vi "Outputs SW Set.vi"(6 "CMD_ACT_Tempplate Data":T1, 7 "Current Time":timestamp format="%<%x %.3X>T", 8 "HW Config":T4={"Ver"=0, "CAN"={"ID"=0, "Bus"=""}, "Output"={"Type"=enum."Counter-Clockwise", "Neutral"=enum."Override to Coast", "Max"={"FWD"=1.0, "REV"=-1.0}, "Min"={"FWD"=0.0, "REV"=0.0}, "OL Ramp Rate (S)"=0.0, "Dead Band"=0.0, "CL Ramp Rate (S)"=0.0}, "CL"={"Gains"={"P"=1.0, "I"=0.01, "D"=0.0, "F"=0.0}, "Error Allowed"=0.0, "I Zone"=0.0, "Peak Out 0-1"=10000.0, "Max I Accu"=-1000.0}, "MM"={"Cruise Velocity"=5000, "Acceleration"=5000}, "TravelLimits"={"Hard"={"FWD Switch Normal"=enum."Normally Open", "FWD On will Zero Encoder "=FALSE, "REV Switch Normal"=enum."Normally Open", "REV On will Zero Encoder "=FALSE}, "Soft"={"FWD"={"Enable"=FALSE, "Counts"=0}, "REV"={"Enable"=FALSE, "Counts"=0}}}, "CurrentLimit"={"Enable"=FALSE, "Current Limit"=0.0, "Threshold Current"=0.0, "Threshold Time"=0.0}} {"CL"."Gains"."F" format="%#.8f"; "CL"."Gains"."D" format="%#.8f"; "CL"."Gains"."I" format="%#.8f"; "CL"."Gains"."P" format="%#.8f"; "Output"."Min"."REV" format="%.2f"; "Output"."Min"."FWD" format="%.2f"; "Output"."Max"."REV" format="%.2f"; "Output"."Max"."FWD" format="%.2f"; "TravelLimits"."Soft"."REV"."Counts" format="%#.0f"; "TravelLimits"."Soft"."FWD"."Counts" format="%#.0f"}, 9 "SW Config":T19={"Ver"=0, "Pivot Arm Position Table"={"Full Back"=0.2, "Full Forward"=0.0, "Amp Score"=0.0, "Pivot Arm Load"=0.0, "Vertical"=0.0, "Trap Score"=0.0}}, 10 "Sensor Values":T22 {"Set"."Mode" items=["PercentOutput"=0, "Position"=1, "Velocity"=2, "Current"=3, "Follower"=5, "MotionProfile"=6, "MotionMagic"=7, "MotionProfileArc"=10, "Disabled"=15]}, 11 "SW Output":T21) -> (3 "SW Output Out":T21)   [LabVIEW 2023, in "Shooter FX_ACT.lvlib"]
uses:
  Shooter FX_ACT.lvlib
  Shared Code/TypeDefs/Cluster_FX Sensor Values.ctl
  Shared Code/TypeDefs/Cluster_FX CloseLoop Values.ctl
  Shared Code/TypeDefs/Cluster_FX Limit Switchs.ctl
  Shared Code/TypeDefs/Cluster_FX Current Values.ctl
  Cluster_HW Output Values.ctl
  Cluster_SW Output Data.ctl
  Cluster_Config SW Values.ctl
  Shared Code/TypeDefs/Cluster_FWD  REV Values.ctl
  Shared Code/TypeDefs/Cluster_PID Gains.ctl
  Shared Code/TypeDefs/Cluster_FX Motion Magic Parameters.ctl
  Shared Code/TypeDefs/Cluser_CAN Data.ctl
  <vilib>/Rock Robotics/WPI/ThirdParty/Phoenix-LabVIEW/Motor Controller/Controls/CTRE_Phoenix_MotorControl_NeutralMode.ctl
  <vilib>/Rock Robotics/WPI/ThirdParty/Phoenix-LabVIEW/Motor Controller/Controls/CTRE_Phoenix_MotorControl_LimitSwitchNormal.ctl
  Shared Code/TypeDefs/Cluser_Hard Limits.ctl
  Shared Code/TypeDefs/Cluser_Enable-Value I32.ctl
  Shared Code/TypeDefs/Cluser_Config_Soft Limits.ctl
  Shared Code/TypeDefs/Cluser_FX Config_Limit Travel.ctl
  Cluster_Config HW Values.ctl
  Shared Code/TypeDefs/Cluser_FX Config_Current Limits.ctl
  Shared Code/TypeDefs/Cluster_FX_HW All Sensor Values.ctl
  <vilib>/Rock Robotics/WPI/ThirdParty/Phoenix-LabVIEW/Motor Controller/Controls/CTRE_Phoenix_MotorControl_ControlMode.ctl
  Shared Code/TypeDefs/Cluster_FX Output Set Values.ctl
  <vilib>/Rock Robotics/WPI/ThirdParty/Phoenix-LabVIEW/Motor Controller/Controls/CTRE_Phoenix_MotorControl_TalonFXInvertType.ctl
  Shared Code/TypeDefs/Cluster_Config FX Motor Output.ctl
  Shared Code/TypeDefs/Cluster_FX SLOT PID Config.ctl
  Shared Code/TypeDefs/Cluster_Pivot Arm Position Table.ctl
  ENUM_CMD_Mode Select.ctl
  Shared Code/TypeDefs/ENUM_Pivot Arm Position Select.ctl
  Cluster_CMD_ACT_Data.ctl
panel:
  # "Tune Output\nto 1023 Max"
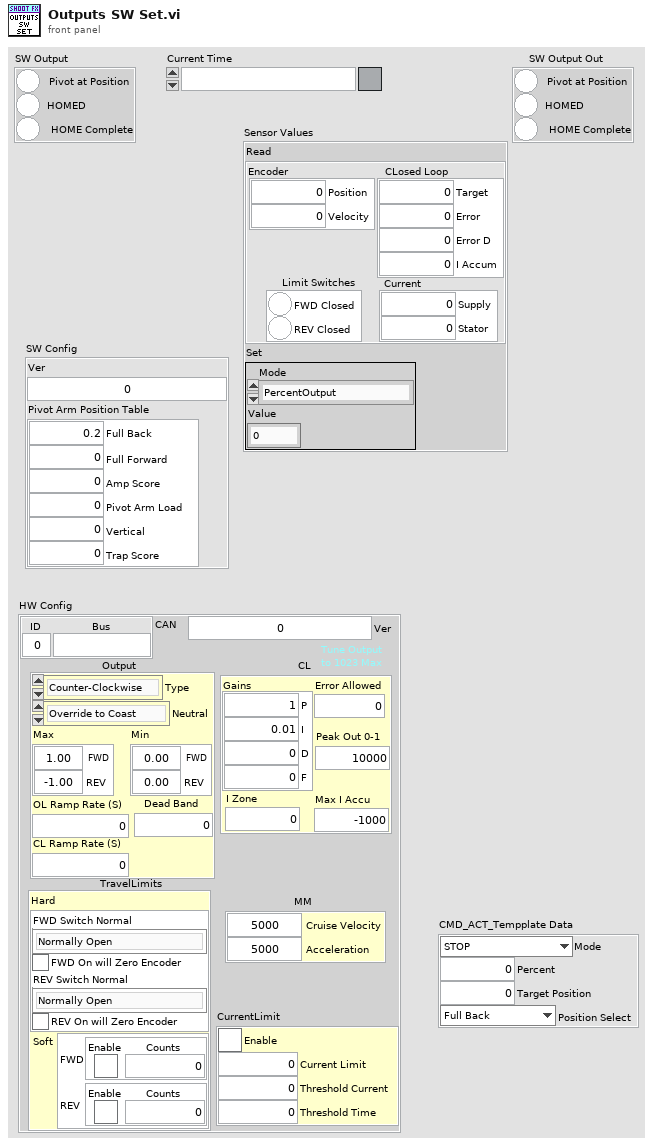
[diagram p1: front panel]
types:
  T1 = typedef "Shooter FX_ACT.lvlib/Cluster_CMD_ACT_Data.ctl" = cluster{"Mode":T2, "Percent":dbl, "Target Position":dbl, "Position Select":T3}
  T2 = typedef "Shooter FX_ACT.lvlib/ENUM_CMD_Mode Select.ctl" = enum16{"STOP", "PercentOut", "Positon Value", "Position Select"}
  T3 = typedef "ENUM_Pivot Arm Position Select.ctl" = enum16{"Full Back", "Full Forward", "Amp Score", "Pivot Arm Load", "Vertical", "Trap Score"}
  T4 = typedef "Shooter FX_ACT.lvlib/Cluster_Config HW Values.ctl" = cluster{"Ver":u64, "CAN":T5, "Output":T6, "CL":T10, "MM":T12, "TravelLimits":T13, "CurrentLimit":T18}
  T5 = typedef "Cluser_CAN Data.ctl" = cluster{"ID":u8, "Bus":string}
  T6 = typedef "Cluster_Config FX Motor Output.ctl" = cluster{"Type":T7, "Neutral":T8, "Max":T9, "Min":T9, "OL Ramp Rate (S)":dbl, "Dead Band":dbl, "CL Ramp Rate (S)":dbl}
  T7 = typedef "CTRE_Phoenix_MotorControl_TalonFXInvertType.ctl" = enum16{"Counter-Clockwise", "Clockwise"}
  T8 = typedef "CTRE_Phoenix_MotorControl_NeutralMode.ctl" = enum8{"EEPROMSetting", "Override to Coast", "Override to Brake"}
  T9 = typedef "Cluster_FWD  REV Values.ctl" = cluster{"FWD":dbl, "REV":dbl}
  T10 = typedef "Cluster_FX SLOT PID Config.ctl" = cluster{"Gains":T11, "Error Allowed":dbl, "I Zone":dbl, "Peak Out 0-1":dbl, "Max I Accu":dbl}
  T11 = typedef "Cluster_PID Gains.ctl" = cluster{"P":dbl, "I":dbl, "D":dbl, "F":dbl}
  T12 = typedef "Cluster_FX Motion Magic Parameters.ctl" = cluster{"Cruise Velocity":i32, "Acceleration":i32}
  T13 = typedef "Cluser_FX Config_Limit Travel.ctl" = cluster{"Hard":T14, "Soft":T16}
  T14 = typedef "Cluser_Hard Limits.ctl" = cluster{"FWD Switch Normal":T15, "FWD On will Zero Encoder ":bool, "REV Switch Normal":T15, "REV On will Zero Encoder ":bool}
  T15 = typedef "CTRE_Phoenix_MotorControl_LimitSwitchNormal.ctl" = enum16{"Normally Open", "Normally Closed", "Disabled"}
  T16 = typedef "Cluser_Config_Soft Limits.ctl" = cluster{"FWD":T17, "REV":T17}
  T17 = typedef "Cluser_Enable-Value I32.ctl" = cluster{"Enable":bool, "Counts":i32}
  T18 = typedef "Cluser_FX Config_Current Limits.ctl" = cluster{"Enable":bool, "Current Limit":dbl, "Threshold Current":dbl, "Threshold Time":dbl}
  T19 = typedef "Shooter FX_ACT.lvlib/Cluster_Config SW Values.ctl" = cluster{"Ver":u64, "Pivot Arm Position Table":T20}
  T20 = typedef "Cluster_Pivot Arm Position Table.ctl" = cluster{"Full Back":dbl, "Full Forward":dbl, "Amp Score":dbl, "Pivot Arm Load":dbl, "Vertical":dbl, "Trap Score":dbl}
  T21 = typedef "Shooter FX_ACT.lvlib/Cluster_SW Output Data.ctl" = cluster{"Pivot at Position":bool, "HOMED":bool, "HOME Complete":bool}
  T22 = typedef "Shooter FX_ACT.lvlib/Cluster_HW Output Values.ctl" = cluster{"Read":T23, "Set":T28}
  T23 = typedef "Cluster_FX_HW All Sensor Values.ctl" = cluster{"Encoder":T24, "CLosed Loop":T25, "Limit Switches":T26, "Current":T27}
  T24 = typedef "Cluster_FX Sensor Values.ctl" = cluster{"Position":i32, "Velocity":i32}
  T25 = typedef "Cluster_FX CloseLoop Values.ctl" = cluster{"Target":dbl, "Error":i32, "Error D":dbl, "I Accum":dbl}
  T26 = typedef "Cluster_FX Limit Switchs.ctl" = cluster{"FWD Closed":bool, "REV Closed":bool}
  T27 = typedef "Cluster_FX Current Values.ctl" = cluster{"Supply":dbl, "Stator":dbl}
  T28 = typedef "Cluster_FX Output Set Values.ctl" = cluster{"Mode":T29, "Value":dbl}
  T29 = typedef "CTRE_Phoenix_MotorControl_ControlMode.ctl" = u16
  T30 = cluster{"Start Time":timestamp, "Prev AT Target Pos":bool, "Home Complete":bool}
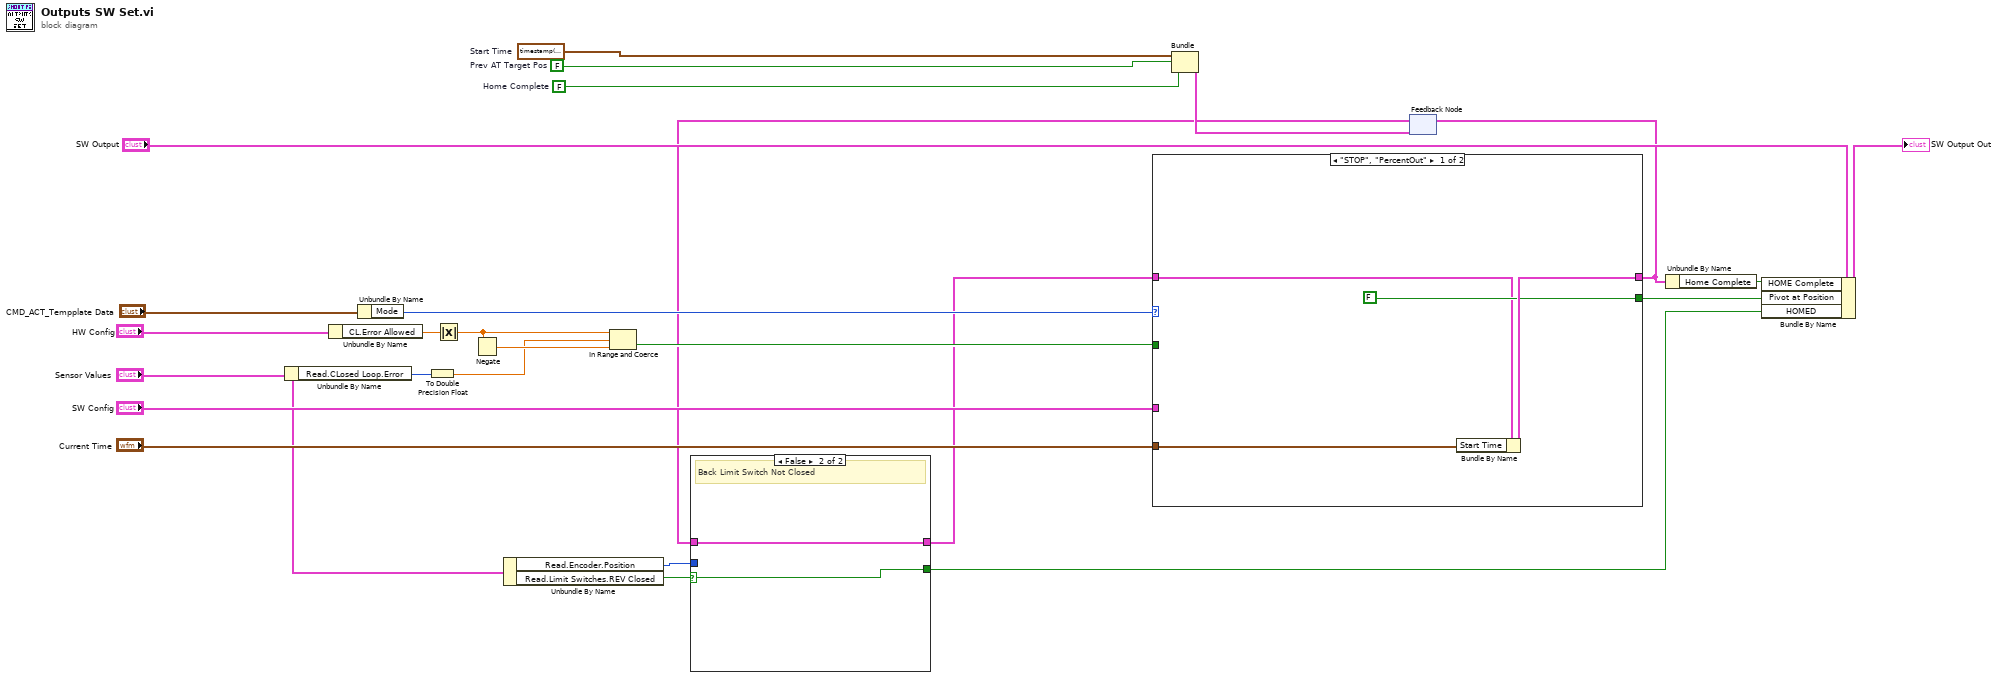
[diagram p0: block diagram]
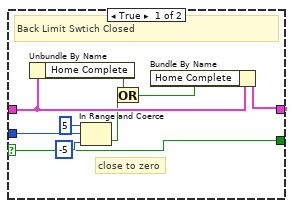
[diagram p2: hidden frame]
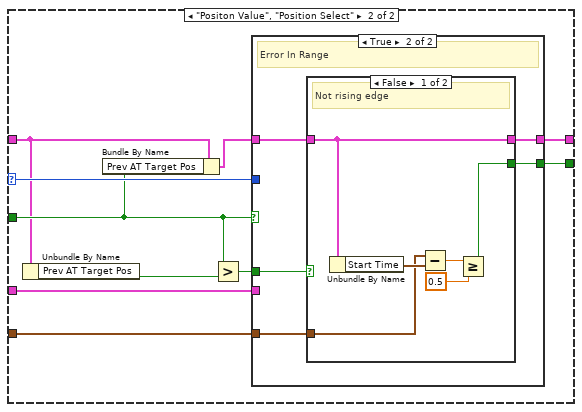
[diagram p3: hidden frame]
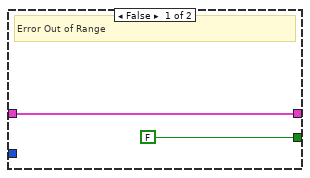
[diagram p4: hidden frame]
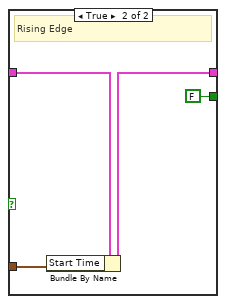
[diagram p5: hidden frame]
diagram:
  w5 = FALSE  # Home Complete
  w10 = FALSE  # Prev AT Target Pos
  w24 = timestamp(0 s since 1904-01-01)  # Start Time
  n1 = Unbundle By Name("Sensor Values") -> ("Read.CLosed Loop.Error"=w19:i32)
  n2 = Unbundle By Name("HW Config") -> ("CL.Error Allowed"=w17:dbl)
  n3 = Unbundle By Name("CMD_ACT_Tempplate Data") -> ("Mode"=w11:T2)
  n4 = To Double Precision Float(number=w19) -> (double precision float=w13:dbl)
  n5 = Absolute Value(x=w17) -> (abs(x)=w16:dbl)
  n6 = Negate(x=w16) -> (-x=w15:dbl)
  n7 = Unbundle By Name("Sensor Values") -> ("Read.Encoder.Position"=w7:i32, "Read.Limit Switches.REV Closed"=w8:bool)
  n8 = In Range and Coerce(upper limit=w16, x=w13, lower limit=w15) -> (In Range?=w18:bool)  [unwired: 1 out]
  n9 = Bundle("Start Time"=w24, "Prev AT Target Pos"=w10, "Home Complete"=w5) -> (w23:T30)  [unwired: 1 in]
  n10 = feedback #1(w23) -> (w4:T30)
  n11 = case shown="False" w8 {
    selector: w8 -> [w28 w37]
    tunnel: w7 -> [w34 _]
    tunnel: [w28 w37] -> w6
    tunnel: w4 -> [w33 w36]
    tunnel: [w35 w36] -> w3
    frame True {
      # "close to zero"
      # "Back Limit Swtich Closed"
      n12 = Unbundle By Name(w33) -> ("Home Complete"=w29:bool)
      n13 = In Range and Coerce(upper limit=5, x=w34, lower limit=-5 ("upper limit")) -> (In Range?=w27:bool)  [unwired: 1 out]
      n14 = Or(x=w29, y=w27) -> (x .or. y?=w30:bool)
      n15 = Bundle By Name(cluster=w33, "Home Complete"=w30) -> (w35:T30)
    }
    frame False {
      # "Back Limit Switch Not Closed"
    }
  }
  n16 = case shown="\"STOP\", \"PercentOut\"" w11 {
    selector: w11 -> [_ w47]
    tunnel: "SW Config" -> [_ w51]
    tunnel: "Current Time" -> [w41 w50]
    tunnel: [w40 w49] -> w2
    tunnel: w18 -> [_ w44]
    tunnel: [FALSE ("Out Data 1") w48] -> w14
    tunnel: w3 -> [w38 w42]
    frame "STOP", "PercentOut" {
      n17 = Bundle By Name(cluster=w38, "Start Time"=w41) -> (w40:T30)
    }
    frame "Positon Value", "Position Select" {
      n18 = Unbundle By Name(w42) -> ("Prev AT Target Pos"=w46:bool)
      n19 = Bundle By Name(cluster=w42, "Prev AT Target Pos"=w44) -> (w43:T30)
      n20 = Greater?(x=w44, y=w46) -> (0:w45:bool)
      n21 = case shown="True" w44 {
        tunnel: w51 -> [_ _]
        tunnel: w43 -> [w52 w58]
        tunnel: [w52 w54] -> w49
        tunnel: w50 -> [_ w56]
        tunnel: [FALSE ("Out Data 1") w57] -> w48
        tunnel: w47 -> [_ _]
        tunnel: w45 -> [_ w55]
        frame False {
          # "Error Out of Range"
        }
        frame True {
          # "Error In Range"
          n22 = case shown="False" w55 {
            tunnel: w58 -> [w59 w67]
            tunnel: [w61 FALSE] -> w57
            tunnel: w56 -> [w60 w65]
            tunnel: [w59 w66] -> w54
            frame False {
              # "Not rising edge"
              n23 = Unbundle By Name(w59) -> ("Start Time"=w64:timestamp)
              n24 = Subtract(x=w60, y=w64) -> (x-y=w63:dbl)
              n25 = Greater Or Equal?(x=w63, y=0.5) -> (x >= y?=w61:bool)
            }
            frame True {
              # "Rising Edge"
              n26 = Bundle By Name(cluster=w67, "Start Time"=w65) -> (w66:T30)
            }
          }
        }
      }
    }
  }
  n27 = feedback-in #1(w2) -> ()
  n28 = Unbundle By Name(w2) -> ("Home Complete"=w1:bool)
  n29 = Bundle By Name(cluster="SW Output", "HOME Complete"=w1, "Pivot at Position"=w14, "HOMED"=w6) -> (→"SW Output Out":T21)
